vi "P4CMD Dialog - File History.vi"(6 "files":string[](array[string]), 7 "fstat info":string, 8 "error in (no error)":errorcluster, 10 "revision string":string, 11 "source control reference in":T1) -> (0 "error out":errorcluster, 5 "file changed?":bool)   [LabVIEW 2017, in "NI_SCC_P4CMD.lvlib"]
uses:
  <vilib>/SourceControl/Providers/P4CMD/NI_SCC_P4CMD.lvlib
  <vilib>/SourceControl/sccapi/SCCAPI Refnum.ctl
  <vilib>/event_ctls.llb/sizeaction.ctl
  <vilib>/event_ctls.llb/panelstate.ctl
  <vilib>/SourceControl/Providers/P4CMD/P4CMD Operations.ctl
  <vilib>/SourceControl/support/SCCSup Message Strings GLBL.vi
  <vilib>/SourceControl/sccapi/NI_SCC.lvlib
  <vilib>/Utility/lvfile.llb/NI_FileType.lvlib
panel:
  in  "History":i32[](listbox)
  in  "Depot file":i32(ring)
  out "File type:":string
  out "Actions in changelist":string
  out "Description of changelist":string
  in  "OK":bool
  in  "Help":bool
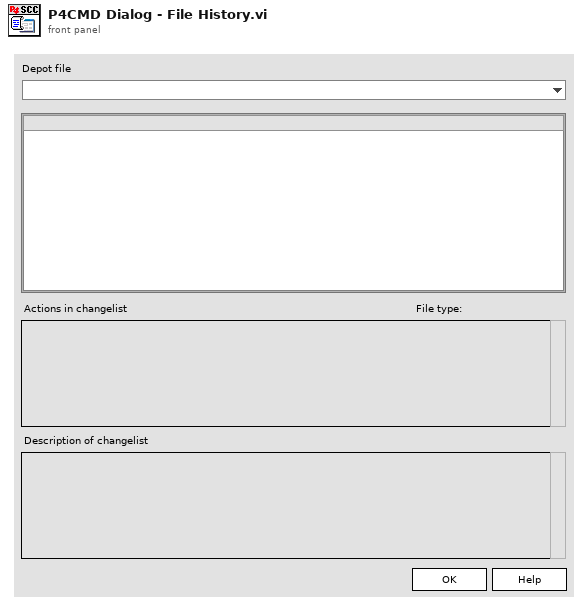
[diagram p1: front panel]
types:
  T1 = typedef "NI_SCC.lvlib/SCCAPI Refnum.ctl" = refnum<k1>
  T2 = enum32{"invalid OS target", "Mac OS", "Windows 3.1", "Windows 95/NT", "Solaris 1", "Solaris 2", "HP-UX", "PowerMAX", "Linux", "Irix", "Rhapsody", "BeOS", "AIX", "OSF1", "VxWorks", "PharLap", "Carbon", "RTX", "Windows x64", "Linux x64"}
  T3 = typedef "sizeaction.ctl" = enum32{"Minimized", "Maximized", "Resized"}
  T4 = typedef "panelstate.ctl" = enum32{"Standard", "Minimized", "Maximized"}
  T5 = typedef "NI_SCC_P4CMD.lvlib/P4CMD Operations.ctl" = enum16{"get all clients", "get all users", "describe changelist", "sync from depot", "open for edit", "submit to depot", "revert", "add to depot", "remove from depot", "print files revisions", "compare client file", "print depot file contents", "list opened files", "get file info", "lock files", "edit changelist spec", "info", "set variables"}
  T6 = enum32{"Invalid", "Standard", "Closed", "Hidden", "Minimized", "Maximized"}
  T7 = typedef "imagedata.ctl" = cluster{"image type":i32, "image depth":i32, "image":u8[], "mask":u8[], "colors":u32[], "Rectangle":cluster{"left":i16, "top":i16, "right":i16, "bottom":i16}}
  T8 = typedef "LVRectTypeDef.ctl" = cluster{"Left":i16, "Top":i16, "Right":i16, "Bottom":i16}
  T9 = enum32{"invalid OS target", "Mac OS", "Windows 3.1", "Windows 95/NT", "Solaris 1", "Solaris 2", "HP-UX", "PowerMAX", "Linux", "Irix", "Rhapsody", "BeOS", "AIX", "OSF1", "VxWorks", "PharLap", "Carbon", "RTX", "Windows x64", "Linux x64", "Mac OS X x64"}
  T10 = typedef "eventvkey.ctl" = enum16{"ASCII", "Enter", "Return", "Shift", "Ctrl", "Alt", "Cmd", "Opt", "Caps", "NumLock", "Clear", "Break", "Up", "Down", "Left", "Right", "Insert", "Delete", "Home", "End", "PageUp", "PageDown", "Escape", "Help", "Pause", "ScrollLock", "F1", "F2", "F3", "F4", "F5", "F6", "F7", "F8", "F9", "F10", "F11", "F12", "F13", "F14", "F15", "F16", "F17", "F18", "F19", "F20", "F21", "F22", "F23", "F24", "Play", "VolumeUp", "VolumeDown", "Mute", "Two Byte Char"}
  T11 = typedef "LVPoint32TypeDef.ctl" = cluster{"Horizontal":i32, "Vertical":i32}
  T12 = typedef "LVRowAndColumnTypeDef.ctl" = cluster{"Row":i32, "Column":i32}
  T13 = typedef "NI_SCC.lvlib/SCCAPI VI Compare Options.ctl" = cluster{"VI Attributes":bool, "Front Panel":bool, "FP position/size":bool, "Block Diagram":bool, "BD cosmetic":bool, "BD position/size":bool}
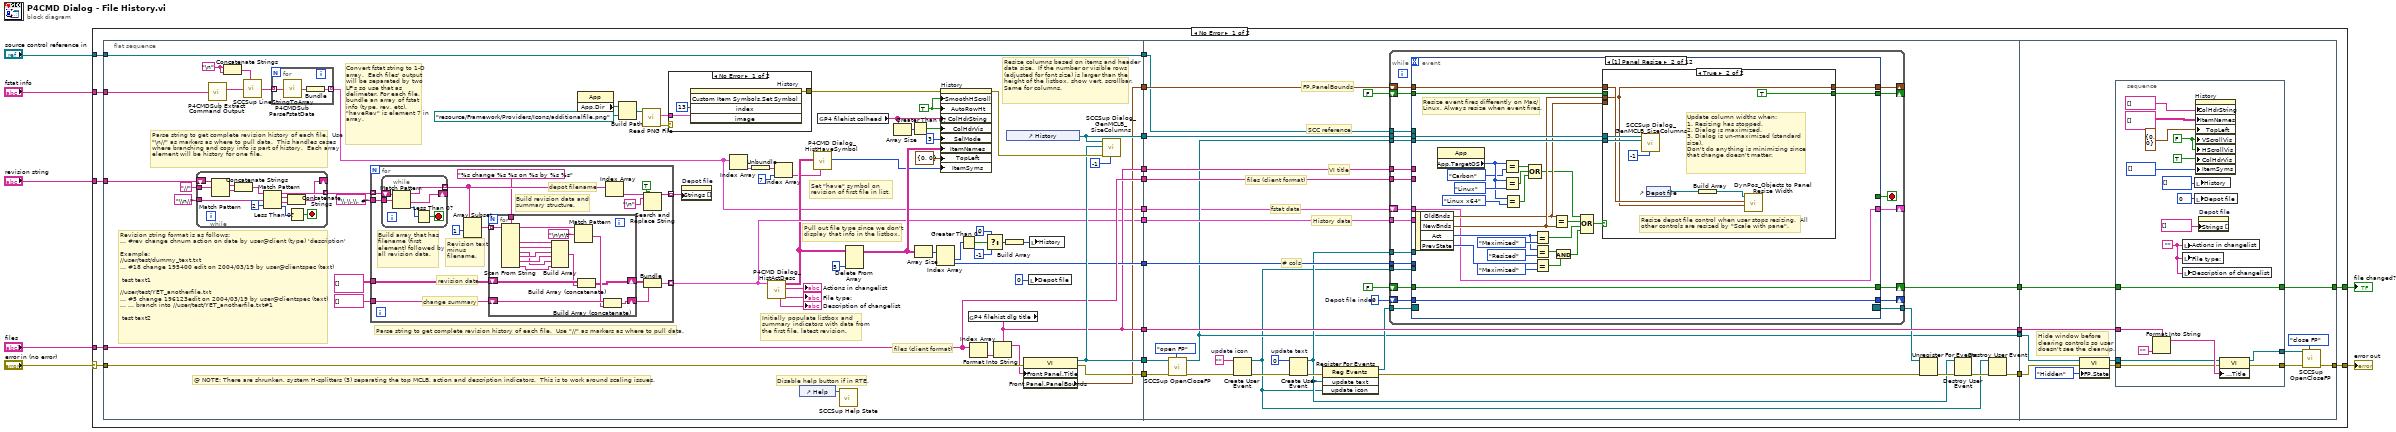
[diagram p0: block diagram]
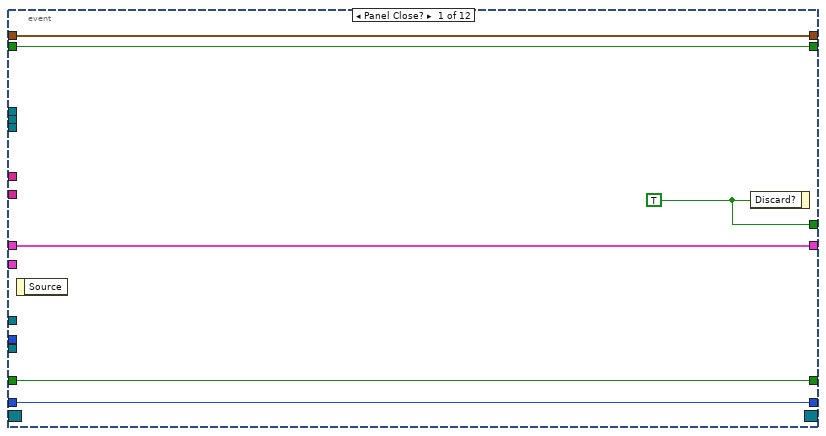
[diagram p3: hidden frame]
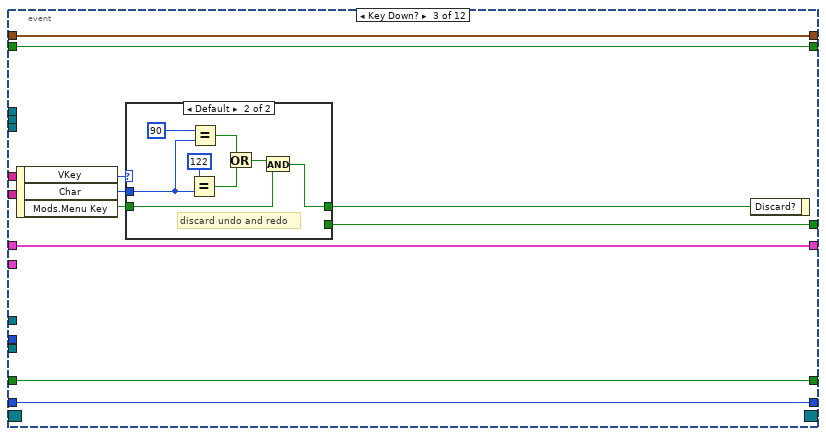
[diagram p6: hidden frame]
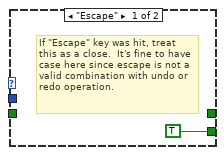
[diagram p7: hidden frame]
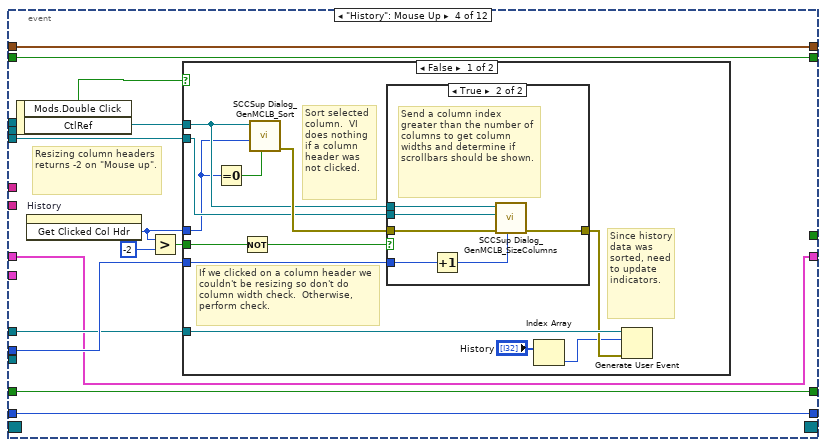
[diagram p8: hidden frame]
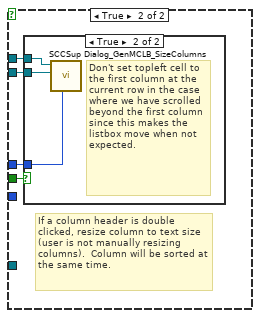
[diagram p10: hidden frame]
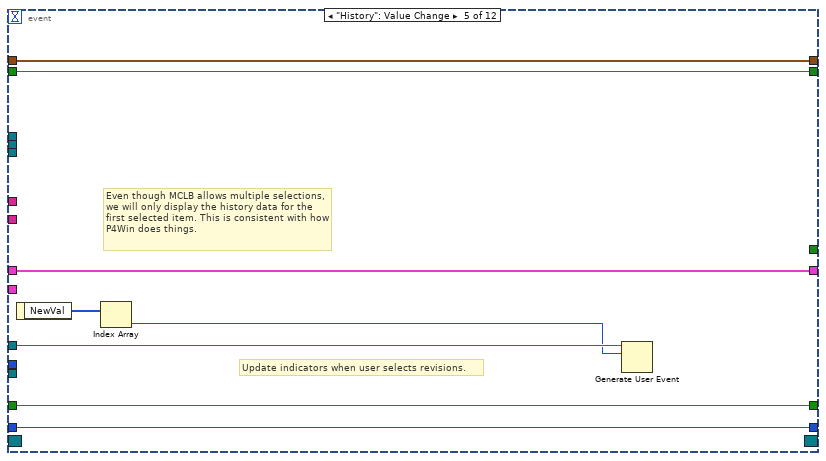
[diagram p12: hidden frame]
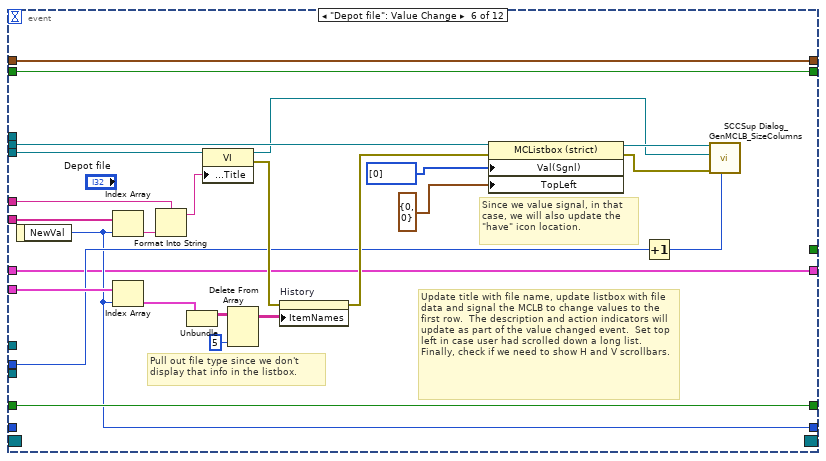
[diagram p13: hidden frame]
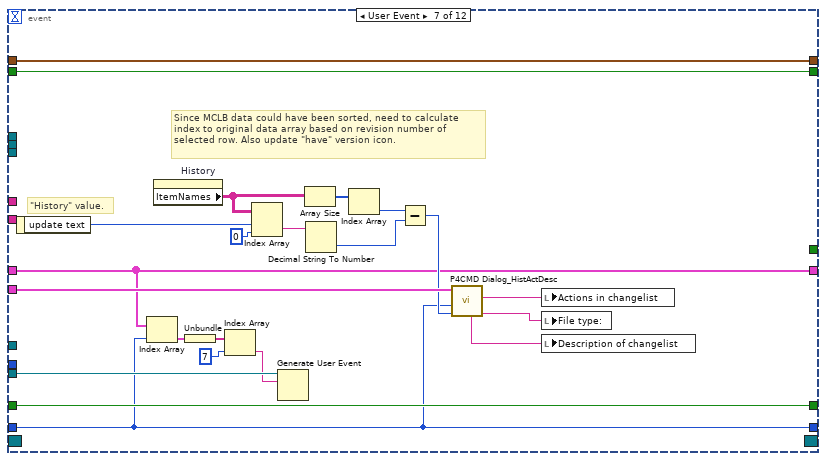
[diagram p14: hidden frame]
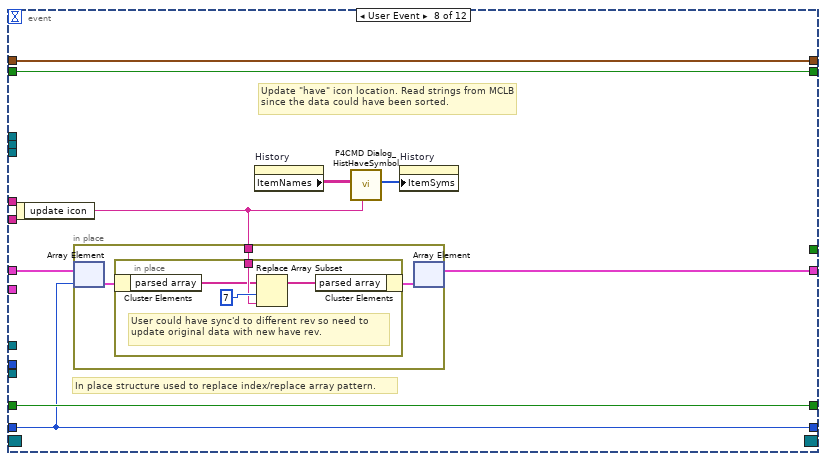
[diagram p15: hidden frame]
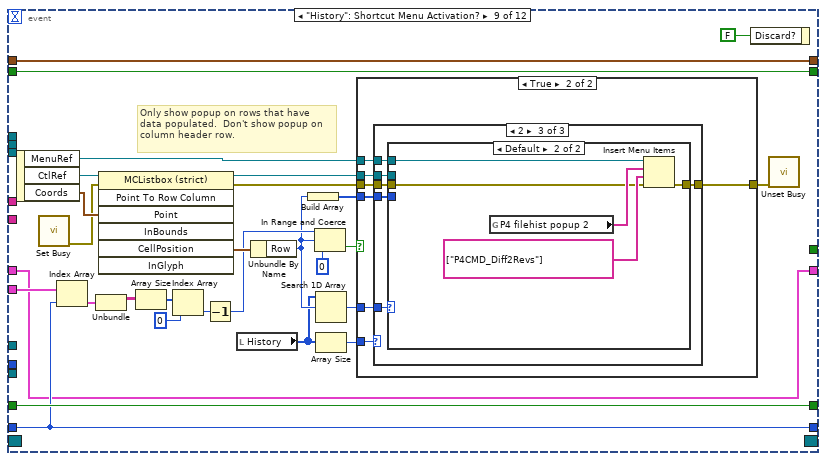
[diagram p16: hidden frame]
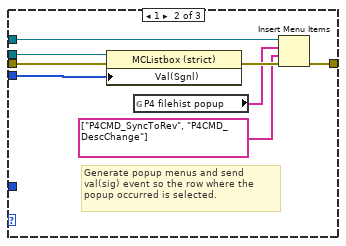
[diagram p19: hidden frame]
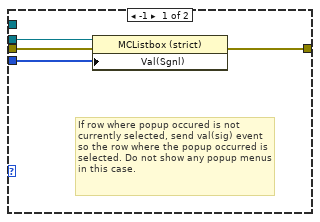
[diagram p20: hidden frame]
diagram:
  n1 = case shown="No Error" "error in (no error)" {
    selector: "error in (no error)" -> [w25 w574]
    tunnel: "revision string" -> [w26 _]
    tunnel: [w22 w574] -> w5
    tunnel: "files" -> [w19 _]
    tunnel: "source control reference in" -> [w13 _]
    tunnel: [w10 _] -> w2
    tunnel: "fstat info" -> [w9 _]
    frame No Error {
      n2 = flat-sequence {
        tunnel: [w82] -> w29
        tunnel: [w83] -> w28
        tunnel: w25 -> [w78]
        tunnel: w26 -> [w60]
        tunnel: [w77] -> w24
        tunnel: [w36] -> w21
        tunnel: [w68] -> w20
        tunnel: w19 -> [w72]
        tunnel: [w72] -> w18
        tunnel: [w64] -> w17
        tunnel: [w64] -> w16
        tunnel: [w56] -> w14
        tunnel: w13 -> [w52]
        tunnel: [w52] -> w12
        tunnel: w9 -> [w39]
        tunnel: [w34] -> w8
        tunnel: [w158] -> w27
        tunnel: w29 -> [w174]
        tunnel: w28 -> [w173]
        tunnel: w24 -> [w172]
        tunnel: [w148] -> w23
        tunnel: w21 -> [w170]
        tunnel: w20 -> [w171]
        tunnel: w18 -> [w169]
        tunnel: w17 -> [w168]
        tunnel: w16 -> [w167]
        tunnel: [w167] -> w15
        tunnel: w14 -> [w166]
        tunnel: w12 -> [w157]
        tunnel: [w155] -> w11
        tunnel: w8 -> [w146]
        tunnel: w27 -> [w549]
        tunnel: w23 -> [w546]
        tunnel: [w551] -> w22
        tunnel: w15 -> [w554]
        tunnel: w11 -> [w545]
        tunnel: [w544] -> w10
        frame #0 {
          w42 = "\n"
          w63 = TRUE ("Smooth Horizontal Scrolling")
          # "Set \"have\" symbol on revision of first file in list."
          # "Revision string format is as follows:\n... #rev change chnum action on date by user@client (type) 'description'\n\nExample:\n//user/test/dummy_text.txt\n... #18 change 195400 edit on 2004/03/19 by user@clientspec (text)\n\n\ttest text1\n\n//user/test/YET_anotherfile.txt\n... #5 change 196123edit on 2004/03/19 by user@clientspec (text)\n... ... branch into //user/test/YET_anotherfile.txt#1\n\n\ttest text2"
          # "Convert fstat string to 1-D array.  Each files' output will be separated by two LF's so use that as delimeter. For each file, bundle an array of fstat info (type, rev, etc). \"haveRev\" is element 7 in array."
          # "@ NOTE: There are shrunken, system H-splitters (3) separating the top MCLB, action and description indicators.  This is to work around scaling issues."
          # "Pull out file type since we don't display that info in the listbox."
          # "Disable help button if in RTE."
          # "files (client format)"
          # "Parse string to get complete revision history of each file.  Use \"//\" as markers as where to pull data."
          # "Parse string to get complete revision history of each file.  Use \"\\n//\" as markers as where to pull data.  This handles cases where branching and copy info is part of history.  Each array element will be history for one file."
          # "Initially populate listbox and summary indicators with data from the first file, latest revision."
          # "Resize columns based on items and header data size.  If the number or visible rows (adjusted for font size) is larger than the height of the listbox, show vert. scrollbar.  Same for columns."
          n3 = while {
            shift-right: [w101] -> _
            shift-left: w60 -> [w107]
            tunnel: "//" ("format string") -> [w105]
            tunnel: [w104] -> w59 mode=indexing
            tunnel: "\\n//" ("format string") -> [w102]
            stop <- w108 stop-if-true
            n4 = Match Pattern(string=w107, regular expression=w105) -> (match substring=w98:string, after substring=w97:string)  [unwired: 1 in, 2 out]
            n5 = Concatenate Strings(w98, w97) -> (w96:string)
            n6 = Match Pattern(string=w96, regular expression=w102, offset (0)=2) -> (before substring=w104:string, match substring=w99:string, after substring=w106:string, offset past match=w100:i32)
            n7 = Concatenate Strings(w99, w106) -> (w101:string)
            n8 = Less Than 0?(x=w100) -> (x < 0?=w108:bool)
          }
          n9 = call <vilib>:"P4CMDSub Extract Command Output.vi"("bundled message"=w39) -> ("command output"=w40:string)  [unwired: 13 in, 1 out]
          n10 = Concatenate Strings(w42, w42) -> (w41:string)
          n11 = call <vilib>:"SCCSup LineStringToArray.vi"("delimiter (Tab)"=w41, "line string"=w40) -> ("line array"=w38:string[])  [unwired: 7 in]
          n12 = for {
            tunnel: w38 -> [w92] mode=indexing
            tunnel: [w90] -> w34 mode=indexing
            n13 = call <vilib>:"P4CMDSub ParseFstatData.vi"("fstat data"=w92) -> ("parsed array"=w91:string[])  [unwired: 4 in]
            n14 = Bundle("parsed array"=w91) -> (w90:cluster{"parsed array":string[]})  [unwired: 1 in]
          }
          n15 = for {
            tunnel: w59 -> [w119] mode=indexing
            tunnel: [w115] -> w75 mode=indexing
            tunnel: "\\.\\.\\. #" ("regular expression") -> [w118]
            tunnel: string[][] [] -> [w114]
            tunnel: string[] [] -> [w113]
            tunnel: [w110] -> w36 mode=indexing
            # "Build revision data and summary structure."
            # "Build array that has filename (first element) followed by all revision data."
            # "Revision text minus filename."
            # "depot filename"
            # "revision data"
            # "change summary"
            n16 = while {
              shift-right: [w125] -> _
              shift-left: w119 -> [w129]
              tunnel: [w128] -> w116 mode=indexing
              tunnel: w118 -> [w124]
              stop <- w127 stop-if-true
              n17 = Match Pattern(string=w129, regular expression=w124) -> (before substring=w128:string, after substring=w125:string, offset past match=w126:i32)  [unwired: 1 in, 1 out]
              n18 = Less Than 0?(x=w126) -> (x < 0?=w127:bool)
            }
            n19 = Array Subset(array=w116, index=1) -> (w122:string[])  [unwired: 1 in]
            n20 = for {
              tunnel: w122 -> [w136] mode=indexing
              shift-right: [w133] -> w112
              shift-left: w114 -> [w145]
              shift-right: [w137] -> w111
              shift-left: w113 -> [w144]
              tunnel: "%s change %s %s on %s by %s %s" ("Format String") -> [w132]
              n21 = Scan From String(format string=w132, input string=w136) -> (remaining string=w131:string, output 1=w143:string, output 2=w142:string, output 3=w138:string, output 4=w140:string, output 5=w139:string, output 6=w130:string)  [unwired: 8 in, 2 out]
              n22 = Build Array(w143, w142, w140, w139, w138, w130) -> (w141:string[])
              n23 = Match Pattern(string=w131, regular expression="\n\n\t") -> (after substring=w134:string)  [unwired: 1 in, 3 out]
              n24 = Build Array (concatenate)(w145, w141) -> (w133:string[][])
              n25 = Build Array (concatenate)(w144, w134) -> (w137:string[])
            }
            n26 = Index Array(array=w116) -> (element=w121:string)  [unwired: 1 in]
            n27 = Search and Replace String(replace all?=TRUE ("replace all? (F)"), input string=w121, search string="\n" ("Line Feed Constant")) -> (result string=w115:string)  [unwired: 5 in, 3 out]
            n28 = Bundle(w112, w111) -> (w110:cluster{string[][], string[]})  [unwired: 1 in]
          }
          n29 = property class="App"() -> ("App.Dir"=w46:path)  [unwired: 2 in, 2 out]
          n30 = Build Path(base path=w46, name or relative path=path "resource/Framework/Providers/Icons/additionalfile.png" ("base path")) -> (appended path=w44:path)
          n31 = call <vilib>:"Read PNG File.vi"("path to PNG file"=w44) -> ("error out"=w43:errorcluster, "image data"=w48:T7)  [unwired: 8 in, 1 out]
          n32 = case shown="No Error" w43 {
            tunnel: [w95 _] -> w49
            tunnel: w48 -> [w94 _]
            frame No Error {
              n33 = invoke on="History" class="MCListbox (strict)" method="Custom Item Symbols.Set Symbol"("index"=13 ("Index"), "image"=w94) -> (error out=w95:errorcluster)  [unwired: 3 in, 4 out]
            }
            frame Error {
              # "If there was a problem reading the custom icon, use default image."
            }
          }
          n34 = property on="Depot file" class="Ring (strict)"("Strings []"=w75) -> ()  [unwired: 2 in, 2 out]
          n35 = Index Array(array=w34) -> (element=w33:cluster{"parsed array":string[]})  [unwired: 1 in]
          n36 = Unbundle(w33) -> ("parsed array"=w32:string[])
          n37 = call <vilib>:"P4CMD Dialog_HistActDesc.vi"("history array"=w36) -> ("file type"=→"File type:":string, "action"=→"Actions in changelist":string, "revision data"=w35:string[][], "description"=→"Description of changelist":string)  [unwired: 7 in]
          n38 = Index Array(array=w32, index=7) -> (element=w30:string)
          n39 = control-ref of="Help"() -> (w58:refnum<vi>)
          n40 = call <vilib>:"P4CMD Dialog_HistHaveSymbol.vi"("have revision"=w30, "history info"=w35) -> ("symbols"=w47:i32[])  [unwired: 9 in]
          n41 = global read "SCCSup Message Strings GLBL.vi" "P4 filehist colhead"() -> (w65:string[])
          n42 = call <vilib>:"SCCSup Help State.vi"("help ref"=w58) -> ()  [unwired: 10 in, 1 out]
          n43 = Delete From Array(array=w35, index (col)=5 ("disabled index (col)")) -> (array with subset deleted=w50:string[][])  [unwired: 2 in, 1 out]
          n44 = Array Size(array=w65) -> (size(s)=w88:i32)
          n45 = Greater Than 0?(x=w88) -> (x > 0?=w66:bool)
          n46 = Array Size(array=w50) -> (size(s)=w69:i32[])
          n47 = Index Array(array=w69) -> (element #1=w51:i32, element #2=w68:i32)  [unwired: 2 in]
          n48 = property on="History" class="MCListbox (strict)"(error in=w49, "SmoothHScroll"=w63, "AutoRowHt"=w63, "ColHdrString"=w65, "ColHdrVis"=w66, "SelMode"=3 ("Selection Mode"), "ItemNames"=w50, "TopLeft"=cluster{"Row":u32, "Column":u32} {"Row"=0, "Column"=0} ("Top Left Visible Cell"), "ItemSyms"=w47) -> (error out=w85:errorcluster)  [unwired: 1 in, 1 out]
          n49 = Greater Than 0?(x=w51) -> (x > 0?=w81:bool)
          n50 = global read "SCCSup Message Strings GLBL.vi" "P4 filehist dlg title"() -> (w64:string)
          n51 = Index Array(array=w72) -> (element=w74:string)  [unwired: 1 in]
          n52 = Select(t=0, s=w81, f=-1 ("index of element")) -> (s? t:f=w89:i32)
          n53 = Format Into String(format string=w64, w74) -> (resulting string=w73:string)  [unwired: 2 in, 1 out]
          n54 = Build Array(w89) -> (w84:i32[])
          n55 = control-ref of="History"() -> (w83:refnum<vi>)
          n56 = property on="Property Node" class="VI"(error in=w78, "Front Panel.Title"=w73) -> (reference out=w82:refnum<vi>, error out=w77:errorcluster, "Front Panel.PanelBounds"=w56:T8)  [unwired: 1 in]
          n57 = local write "Depot file"(0 ("Depot file")) -> ()
          n58 = local write "History"(w84) -> ()
          n59 = call <vilib>:"SCCSup Dialog_GenMCLB_SizeColumns.vi"("column index"=-1, "error in (no error)"=w85, "VI Refnum"=w82, "Multicolumn Listbox"=w83) -> ()  [unwired: 6 in, 2 out]
        }
        frame #1 {
          w152 = ""  # update icon
          w153 = 0  # update text
          w154 = 0  # Depot file index
          # "SCC reference"
          # "# cols"
          # "fstat data"
          # "History data"
          # "VI title"
          # "FP.PanelBounds"
          # "files (client format)"
          n60 = call <vilib>:"SCCSup OpenCloseFP.vi"("function"=enum16{"open FP", "close FP"}."open FP", "error in (no error)"=w172, "VI Refnum in"=w174) -> ("error out"=w150:errorcluster, "VI Refnum out"=w158:refnum<vi>)  [unwired: 7 in]
          n61 = Create User Event(user event datatype=w152, error in=w150) -> (user event=w147:refnum<user-event>, error out=w151:errorcluster)
          n62 = Create User Event(user event datatype=w153, error in=w151) -> (user event=w159:refnum<user-event>, error out=w164:errorcluster)
          n63 = register-events(error in=w164, w159, w147) -> (reference out=w163:refnum<event-registration>, error out=w161:errorcluster)  [unwired: 1 in]
          n64 = while {
            tunnel: w158 -> [w195]
            tunnel: w173 -> [w196]
            tunnel: w171 -> [w194]
            tunnel: w170 -> [w193]
            tunnel: w169 -> [w192]
            tunnel: w168 -> [w191]
            shift-right: [w187] -> _
            shift-left: w166 -> [w190]
            shift-right: [w189] -> _
            shift-left: FALSE -> [w188]
            tunnel: w163 -> [w186]
            tunnel: [w185] -> w162
            tunnel: w159 -> [w184]
            tunnel: w157 -> [w183]
            shift-right: [w181] -> w155
            shift-left: FALSE -> [w182]
            shift-right: [w179] -> _
            shift-left: w154 -> [w180]
            tunnel: w147 -> [w178]
            shift-right: [w176] -> _
            shift-left: w146 -> [w177]
            stop <- w197 stop-if-true
            n65 = event shown="[1] Panel Resize" {
              selector: w186 -> [_ _ _ _ _ _ _ _ _ _ _ _]
              dyn-events: [_ _ _ _ _ _ _ _ _ _ _ _] -> w185
              timeout: _ -> [_ _ _ _ _ _ _ _ _ _ _ _]
              tunnel: [w203 _ w255 _ _ _ _ _ _ w439 "OK" _] -> w197
              tunnel: w196 -> [_ w233 _ _ _ w328 _ _ _ _ _ _]
              tunnel: w195 -> [_ w232 _ w277 _ w338 _ _ _ _ _ _]
              tunnel: w194 -> [_ _ _ w276 _ w319 _ _ _ _ _ _]
              tunnel: w193 -> [_ _ _ _ _ w331 w359 _ w396 _ _ _]
              tunnel: w192 -> [_ _ _ _ _ w339 _ _ _ w453 _ _]
              tunnel: w191 -> [_ _ _ _ _ w336 _ _ _ _ _ _]
              tunnel: w190 -> [w202 w221 w254 w273 w315 w334 w353 w370 w406 w460 w534 w540]
              tunnel: [w201 w218 w253 w274 w314 w333 w352 w369 w405 w459 w533 w539] -> w189
              tunnel: w188 -> [w201 w217 w253 w274 w314 w333 w352 w369 w405 w459 w533 w539]
              tunnel: [w202 w216 w254 w273 w315 w334 w353 w370 w406 w460 w534 w540] -> w187
              tunnel: w184 -> [_ _ _ w272 w313 _ _ _ _ _ _ _]
              tunnel: w183 -> [_ _ _ _ _ _ _ _ _ w448 _ _]
              tunnel: w182 -> [w200 w212 w252 w271 w311 w329 w351 w371 w385 w447 w532 w538]
              tunnel: [w200 w212 w252 w271 w311 w329 w351 w371 w385 w446 w532 w538] -> w181
              tunnel: w180 -> [w199 w211 w251 w270 w310 _ w343 w364 w384 w443 w531 w537]
              tunnel: [w199 w211 w251 w270 w310 w317 w343 w364 w384 w443 w531 w537] -> w179
              tunnel: w178 -> [_ _ _ _ _ _ w348 _ _ w442 _ _]
              tunnel: w177 -> [w198 w210 w250 w269 w308 w316 w341 w365 w383 w441 w530 w536]
              tunnel: [w198 w210 w250 w269 w308 w316 w341 w363 w383 w441 w530 w536] -> w176
              event Panel Close? {
                w203 = TRUE
                n66 = event-data() -> ()  [unwired: 1 in, 1 out]
                n67 = event-data ("Event Filter Node")("Discard?"=w203) -> ()  [unwired: 1 in, 1 out]
              }
              event Panel Resize {
                # "Resize event fires differently on Mac/Linux. Always resize when event fires."
                n68 = event-data() -> ("OldBnds"=w219:T8, "NewBnds"=w220:T8, "Act"=w226:T3, "PrevState"=w228:T4)  [unwired: 1 in]
                n69 = property class="App"() -> ("App.TargetOS"=w207:T9)  [unwired: 2 in, 2 out]
                n70 = Equal?(x=w207, y=T2."Carbon" ("Application:Target:Operating System")) -> (x = y?=w214:bool)
                n71 = Equal?(x=w207, y=T2."Linux" ("Application:Target:Operating System")) -> (x = y?=w208:bool)
                n72 = Equal?(x=w207, y=T2."Linux x64" ("Application:Target:Operating System")) -> (x = y?=w205:bool)
                n73 = Compound Arithmetic op=OR(w214, w208, w205) -> (w213:bool)
                n74 = Equal?(x=w226, y=sizeaction."Maximized") -> (x = y?=w229:bool)
                n75 = Equal?(x=w226, y=sizeaction."Resized") -> (x = y?=w224:bool)
                n76 = Equal?(x=w228, y=panelstate."Maximized" ("PrevState")) -> (x = y?=w223:bool)
                n77 = Equal?(x=w219, y=w220) -> (x = y?=w215:bool)
                n78 = And(x=w224, y=w223) -> (x .and. y?=w222:bool)
                n79 = Compound Arithmetic op=OR(w213, w215, w229, w222) -> (w230:bool)
                n80 = case shown="True" w230 {
                  tunnel: w233 -> [_ w249]
                  tunnel: w232 -> [_ w248]
                  tunnel: w221 -> [w238 w244]
                  tunnel: w220 -> [_ w243]
                  tunnel: w219 -> [w237 _]
                  tunnel: [w236 TRUE] -> w218
                  tunnel: w217 -> [w235 _]
                  tunnel: [w234 w243] -> w216
                  frame False {
                    # "Save panel bound after first resize so when resize stops, we can do a correct delta. Once we get the bounds, just pass value through all cases."
                    n81 = case shown="True" w235 {
                      selector: w235 -> [w240 _]
                      tunnel: w238 -> [w239 _]
                      tunnel: w237 -> [_ w241]
                      tunnel: [w240 _] -> w236
                      tunnel: [w239 w241] -> w234
                      frame False {
                      }
                      frame True {
                      }
                    }
                  }
                  frame True {
                    # "Update column widths when:\n1. Resizing has stopped.\n2. Dialog is maximized.\n3. Dialog is un-maximized (standard size).\nDon't do anything is minimizing since that change doesn't matter."
                    # "Resize depot file control when user stops resizing.  All other controls are resized by \"Scale with pane\"."
                    n82 = call <vilib>:"SCCSup Dialog_GenMCLB_SizeColumns.vi"("column index"=-1, "VI Refnum"=w248, "Multicolumn Listbox"=w249) -> ()  [unwired: 7 in, 2 out]
                    n83 = control-ref of="Depot file"() -> (w245:refnum<vi>)
                    n84 = Build Array(w245) -> (w246:refnum<vi>[])
                    n85 = call <vilib>:"DynPos_Objects to Panel Resize Width.vi"("NewBnds"=w243, "OldBnds"=w244, "GObj Refnums"=w246) -> ()  [unwired: 8 in, 1 out]
                  }
                }
              }
              event Key Down? {
                n86 = event-data() -> ("VKey"=w256:T10, "Char"=w259:i16, "Mods.Menu Key"=w258:bool)  [unwired: 1 in]
                n87 = case shown="Default" w256 {
                  tunnel: w259 -> [_ w263]
                  tunnel: w258 -> [_ w262]
                  tunnel: [_ w261] -> w257
                  tunnel: [TRUE _] -> w255
                  frame "Escape" {
                    # "If \"Escape\" key was hit, treat this as a close.  It's fine to have case here since escape is not a valid combination with undo or redo operation."
                  }
                  frame Default {
                    # "discard undo and redo"
                    n88 = Equal?(x=i16 122, y=w263) -> (x = y?=w266:bool)
                    n89 = Equal?(x=i16 90, y=w263) -> (x = y?=w265:bool)
                    n90 = Or(x=w265, y=w266) -> (x .or. y?=w264:bool)
                    n91 = And(x=w264, y=w262) -> (x .and. y?=w261:bool)
                  }
                }
                n92 = event-data ("Event Filter Node")("Discard?"=w257) -> ()  [unwired: 1 in, 1 out]
              }
              event "History": Mouse Up {
                # "Resizing column headers returns -2 on \"Mouse up\"."
                n93 = event-data() -> ("Mods.Double Click"=w275:bool, "CtlRef"=w281:refnum<vi>)  [unwired: 1 in]
                n94 = invoke on="History" class="MCListbox (strict)" method="Get Clicked Col Hdr"() -> ("Get Clicked Column Header"=w279:i32)  [unwired: 3 in, 2 out]
                n95 = Greater?(x=w279, y=-2) -> (0:w278:bool)
                n96 = case shown="False" w275 {
                  tunnel: w281 -> [w288 w304]
                  tunnel: w279 -> [w283 w303]
                  tunnel: w278 -> [w293 w302]
                  tunnel: w277 -> [w289 w301]
                  tunnel: w276 -> [w291 _]
                  tunnel: w272 -> [w287 _]
                  frame False {
                    # "Since history data was sorted, need to update indicators."
                    # "Sort selected column.  VI does nothing if a column header was not clicked."
                    # "If we clicked on a column header we couldn't be resizing so don't do column width check.  Otherwise, perform check."
                    n97 = Equal To 0?(x=w283) -> (x = 0?=w282:bool)
                    n98 = Not(x=w293) -> (.not. x?=w292:bool)
                    n99 = call <vilib>:"SCCSup Dialog_GenMCLB_Sort.vi"("treat as number?"=w282, "Clicked Col Hdr"=w283, "MCListbox Refnum"=w288) -> ("error out"=w290:errorcluster)  [unwired: 8 in]
                    n100 = case shown="True" w292 {
                      tunnel: w288 -> [_ w300]
                      tunnel: w289 -> [_ w299]
                      tunnel: w291 -> [_ w297]
                      tunnel: w290 -> [w294 w296]
                      tunnel: [w294 w295] -> w286
                      frame False {
                      }
                      frame True {
                        # "Send a column index greater than the number of columns to get column widths and determine if scrollbars should be shown."
                        n101 = Increment(x=w297) -> (x+1=w298:i32)
                        n102 = call <vilib>:"SCCSup Dialog_GenMCLB_SizeColumns.vi"("column index"=w298, "error in (no error)"=w296, "VI Refnum"=w299, "Multicolumn Listbox"=w300) -> ("error out"=w295:errorcluster)  [unwired: 6 in, 1 out]
                      }
                    }
                    n103 = Index Array(array="History") -> (element=w284:i32)  [unwired: 1 in]
                    n104 = Generate User Event(user event=w287, event data cluster=w284, error in=w286) -> ()  [unwired: 1 in, 2 out]
                  }
                  frame True {
                    # "If a column header is double clicked, resize column to text size (user is not manually resizing columns).  Column will be sorted at the same time."
                    n105 = case shown="True" w302 {
                      tunnel: w303 -> [_ w307]
                      tunnel: w304 -> [_ w306]
                      tunnel: w301 -> [_ w305]
                      frame False {
                      }
                      frame True {
                        # "Don't set topleft cell to the first column at the current row in the case where we have scrolled beyond the first column since this makes the listbox move when not expected."
                        n106 = call <vilib>:"SCCSup Dialog_GenMCLB_SizeColumns.vi"("column index"=w307, "VI Refnum"=w305, "Multicolumn Listbox"=w306) -> ()  [unwired: 7 in, 2 out]
                      }
                    }
                  }
                }
              }
              event "History": Value Change {
                # "Even though MCLB allows multiple selections, we will only display the history data for the first selected item. This is consistent with how P4Win does things."
                # "Update indicators when user selects revisions."
                n107 = event-data() -> ("NewVal"=w312:i32[])  [unwired: 1 in]
                n108 = Index Array(array=w312) -> (element=w309:i32)  [unwired: 1 in]
                n109 = Generate User Event(user event=w313, event data cluster=w309) -> ()  [unwired: 2 in, 2 out]
              }
              event "Depot file": Value Change {
                # "Since we value signal, in that case, we will also update the \"have\" icon location."
                # "Pull out file type since we don't display that info in the listbox."
                # "Update title with file name, update listbox with file data and signal the MCLB to change values to the first row.  The description and action indicators will update as part of the value changed event.  Set top left in case user had scrolled down a long list. Finally, check if we need to show H and V scrollbars."
                n110 = event-data() -> ("NewVal"=w317:i32)  [unwired: 1 in]
                n111 = Index Array(array=w339, index=w317) -> (element=w340:string)
                n112 = Index Array(array=w331, index=w317) -> (element=w332:cluster{string[][], string[]})
                n113 = Format Into String(format string=w336, w340) -> (resulting string=w337:string)  [unwired: 2 in, 1 out]
                n114 = Unbundle(w332) -> (w330:string[][])  [unwired: 1 out]
                n115 = property on="Property Node" class="VI"(reference=w338, "Front Panel.Title"=w337) -> (reference out=w320:refnum<vi>, error out=w325:errorcluster)  [unwired: 1 in]
                n116 = Delete From Array(array=w330, index (col)=5 ("disabled index (col)")) -> (array with subset deleted=w318:string[][])  [unwired: 2 in, 1 out]
                n117 = property on="History" class="MCListbox (strict)"(error in=w325, "ItemNames"=w318) -> (error out=w326:errorcluster)  [unwired: 1 in, 1 out]
                n118 = property on="Property Node" class="MCListbox (strict)"(reference=w328, error in=w326, "Val(Sgnl)"=i32[] [0] ("History"), "TopLeft"=cluster{"Row":u32, "Column":u32} {"Row"=0, "Column"=0} ("Top Left Visible Cell")) -> (reference out=w322:refnum<vi>, error out=w321:errorcluster)
                n119 = Increment(x=w319) -> (x+1=w323:i32)
                n120 = call <vilib>:"SCCSup Dialog_GenMCLB_SizeColumns.vi"("column index"=w323, "error in (no error)"=w321, "VI Refnum"=w320, "Multicolumn Listbox"=w322) -> ()  [unwired: 6 in, 2 out]
              }
              event User Event {
                # "\"History\" value."
                # "Since MCLB data could have been sorted, need to calculate index to original data array based on revision number of selected row. Also update \"have\" version icon."
                n121 = event-data() -> ("update text"=w354:i32)  [unwired: 1 in]
                n122 = Index Array(array=w341, index=w343) -> (element=w346:cluster{"parsed array":string[]})
                n123 = property on="History" class="MCListbox (strict)"() -> ("ItemNames"=w350:string[][])  [unwired: 2 in, 2 out]
                n124 = Unbundle(w346) -> ("parsed array"=w345:string[])
                n125 = Index Array(array=w345, index=7) -> (element=w342:string)
                n126 = Index Array(array=w350, index (row)=w354, index (col)=0 ("disabled index (col)")) -> (element=w357:string)
                n127 = Generate User Event(user event=w348, event data cluster=w342) -> ()  [unwired: 2 in, 2 out]
                n128 = Array Size(array=w350) -> (size(s)=w356:i32[])
                n129 = Decimal String To Number(string=w357) -> (number=w355:i32)  [unwired: 2 in, 1 out]
                n130 = Index Array(array=w356) -> (element=w349:i32)  [unwired: 1 in]
                n131 = Subtract(x=w349, y=w355) -> (x-y=w347:i32)
                n132 = call <vilib>:"P4CMD Dialog_HistActDesc.vi"("revision index (0)"=w347, "depot file index (0)"=w343, "history array"=w359) -> ("file type"=w361:string, "action"=w362:string, "description"=w360:string)  [unwired: 5 in, 1 out]
                n133 = local write "Actions in changelist"(w362) -> ()
                n134 = local write "File type:"(w361) -> ()
                n135 = local write "Description of changelist"(w360) -> ()
              }
              event User Event {
                # "In place structure used to replace index/replace array pattern."
                # "Update \"have\" icon location. Read strings from MCLB since the data could have been sorted."
                n136 = event-data() -> ("update icon"=w366:string)  [unwired: 1 in]
                n137 = in-place {
                  in-place-border: w366 -> [w374]
                  n138 = in-place-array #1(w365, w364) -> (w373:cluster{"parsed array":string[]})
                  n139 = in-place {
                    in-place-border: w374 -> [w377]
                    # "User could have sync'd to different rev so need to update original data with new have rev."
                    n140 = in-place-cluster #2(w373) -> ("parsed array"=w376:string[])
                    n141 = Replace Array Subset(array=w376, new element=w377, index=7) -> (w375:string[])
                    n142 = in-place-cluster #2("parsed array"=w375) -> (w372:cluster{"parsed array":string[]})
                  }
                  n143 = in-place-array #1(w372) -> (w363:cluster{"parsed array":string[]}[])  [unwired: 1 out]
                }
                n144 = property on="History" class="MCListbox (strict)"() -> ("ItemNames"=w367:string[][])  [unwired: 2 in, 2 out]
                n145 = call <vilib>:"P4CMD Dialog_HistHaveSymbol.vi"("have revision"=w366, "history info"=w367) -> ("symbols"=w368:i32[])  [unwired: 9 in]
                n146 = property on="History" class="MCListbox (strict)"("ItemSyms"=w368) -> ()  [unwired: 2 in, 2 out]
              }
              event "History": Shortcut Menu Activation? {
                # "Only show popup on rows that have data populated.  Don't show popup on column header row."
                n147 = event-data() -> ("MenuRef"=w389:refnum<k9>, "CtlRef"=w404:refnum<vi>, "Coords"=w403:T11)  [unwired: 1 in]
                n148 = call <vilib>:"Set Busy.vi"() -> ("error out"=w402:errorcluster)  [unwired: 10 in, 1 out]
                n149 = Index Array(array=w396, index=w384) -> (element=w401:cluster{string[][], string[]})
                n150 = Unbundle(w401) -> (w400:string[][])  [unwired: 1 out]
                n151 = invoke class="MCListbox (strict)" method="Point To Row Column"(reference=w404, error in=w402, "Point"=w403) -> (reference out=w390:refnum<vi>, error out=w391:errorcluster, "CellPosition"=w395:T12)  [unwired: 4 in, 4 out]
                n152 = Array Size(array=w400) -> (size(s)=w399:i32[])
                n153 = Index Array(array=w399, index=0) -> (element=w398:i32)
                n154 = Decrement(x=w398) -> (x-1=w394:i32)
                n155 = local read "History"() -> (w380:i32[])
                n156 = Unbundle By Name(w395) -> ("Row"=w381:i32)
                n157 = Build Array(w381) -> (w388:i32[])
                n158 = In Range and Coerce(upper limit=w394, x=w381, lower limit=0 ("upper limit")) -> (In Range?=w392:bool)  [unwired: 1 out]
                n159 = Search 1D Array(1D array=w380, element=w381) -> (index of element=w379:i32)  [unwired: 1 in]
                n160 = Array Size(array=w380) -> (size(s)=w382:i32)
                n161 = case shown="True" w392 {
                  tunnel: w391 -> [w407 w414]
                  tunnel: w390 -> [_ w413]
                  tunnel: w389 -> [_ w411]
                  tunnel: w388 -> [_ w412]
                  tunnel: [w407 w410] -> w387
                  tunnel: w382 -> [_ w409]
                  tunnel: w379 -> [_ w408]
                  frame False {
                  }
                  frame True {
                    n162 = case shown="2" w409 {
                      tunnel: w414 -> [w415 w423 w427]
                      tunnel: w413 -> [_ w422 w425]
                      tunnel: w412 -> [_ w421 w424]
                      tunnel: w411 -> [_ w420 w429]
                      tunnel: [w415 w418 w428] -> w410
                      tunnel: w408 -> [_ _ w426]
                      frame 0, Default {
                      }
                      frame 1 {
                        # "Generate popup menus and send val(sig) event so the row where the popup occurred is selected."
                        n163 = property class="MCListbox (strict)"(reference=w422, error in=w423, "Val(Sgnl)"=w421) -> (error out=w419:errorcluster)  [unwired: 1 out]
                        n164 = global read "SCCSup Message Strings GLBL.vi" "P4 filehist popup"() -> (w416:string[])
                        n165 = Insert Menu Items(6:w419, 7:string[] ["P4CMD_SyncToRev", "P4CMD_DescChange"] ("item names"), 8:w416, 9:w420) -> (0:w418:errorcluster)  [unwired: 2 in, 2 out]
                      }
                      frame 2 {
                        n166 = case shown="Default" w426 {
                          tunnel: w429 -> [_ w438]
                          tunnel: [w430 w437] -> w428
                          tunnel: w427 -> [w432 w434]
                          tunnel: w425 -> [w433 _]
                          tunnel: w424 -> [w431 _]
                          frame -1 {
                            # "If row where popup occured is not currently selected, send val(sig) event so the row where the popup occurred is selected. Do not show any popup menus in this case."
                            n167 = property class="MCListbox (strict)"(reference=w433, error in=w432, "Val(Sgnl)"=w431) -> (error out=w430:errorcluster)  [unwired: 1 out]
                          }
                          frame Default {
                            n168 = global read "SCCSup Message Strings GLBL.vi" "P4 filehist popup 2"() -> (w435:string[])
                            n169 = Insert Menu Items(6:w434, 7:string[] ["P4CMD_Diff2Revs"] ("item names"), 8:w435, 9:w438) -> (0:w437:errorcluster)  [unwired: 2 in, 2 out]
                          }
                        }
                      }
                    }
                  }
                }
                n170 = event-data("Discard?"=FALSE) -> ()  [unwired: 1 in, 1 out]
                n171 = call <vilib>:"Unset Busy.vi"("error in (no error)"=w387) -> ()  [unwired: 10 in, 1 out]
              }
              event "History": Shortcut Menu Selection (User) {
                # "Display any errors.  Error is not fatal to this dialog, so we continue."
                n172 = event-data() -> ("ItemTag"=w454:string, "CtlRef"=w458:refnum<vi>, "Coords"=w457:T11)  [unwired: 1 in]
                n173 = call <vilib>:"Set Busy.vi"() -> ("error out"=w456:errorcluster)  [unwired: 10 in, 1 out]
                n174 = invoke class="MCListbox (strict)" method="Point To Row Column"(reference=w458, error in=w456, "Point"=w457) -> (error out=w450:errorcluster, "CellPosition"=w455:T12)  [unwired: 4 in, 5 out]
                n175 = for {
                  tunnel: w453 -> [w462] mode=indexing
                  tunnel: [w461] -> w449 mode=indexing
                  n176 = call <vilib>:"Command Line String To Path.vi"("string"=w462) -> ("path"=w461:path)
                }
                n177 = property on="History" class="MCListbox (strict)"(error in=w450) -> ("ItemNames"=w452:string[][])  [unwired: 1 in, 2 out]
                n178 = Unbundle By Name(w455) -> ("Row"=w451:i32)
                n179 = local read "History"() -> (w440:i32[])
                n180 = case shown="\"P4CMD_Diff2Revs\"" w454 {
                  tunnel: w452 -> [w472 w479 w497]
                  tunnel: w451 -> [w471 w475 _]
                  tunnel: w449 -> [w468 w484 w499]
                  tunnel: [w463 w478 w498] -> w445
                  tunnel: w448 -> [w467 w481 w501]
                  tunnel: w447 -> [w466 _ w502]
                  tunnel: [w466 TRUE w502] -> w446
                  tunnel: w443 -> [_ w477 w500]
                  tunnel: w442 -> [_ w476 _]
                  tunnel: w440 -> [_ _ w496]
                  tunnel: [_ _ w491] -> w439
                  frame "P4CMD_DescChange", Default {
                    # "Files input (and even SCC ref) is not needed, but wire anyway."
                    n181 = Index Array(array=w472, index (row)=w471, index (col)=1 ("disabled index (col)")) -> (element=w469:string)
                    n182 = call <vilib>:"P4CMD Execute Command.vi"("optional operation parameters"=w469, "p4 operation"=P4CMD_Operations."describe changelist", "files"=w468, "source control reference in"=w467) -> ("error out"=w464:errorcluster, "command information"=w465:string)  [unwired: 5 in, 1 out]
                    n183 = call <vilib>:"P4CMD Dialog_HistDispChangelist.vi"("error in (no error)"=w464, "changelist description"=w465) -> ("error out"=w463:errorcluster)  [unwired: 9 in]
                  }
                  frame "P4CMD_SyncToRev" {
                    # "Since we force a sync during a get, notify user that file may have changed."
                    # "Get currently active depot file's client representation at selected revision."
                    n184 = Index Array(array=w479, index (row)=w475, index (col)=0 ("disabled index (col)")) -> (element=w474:string)
                    n185 = Concatenate Strings("#" ("string"), w474) -> (w486:string)
                    n186 = Array Subset(array=w484, index=w477, length=1) -> (w483:path[])
                    n187 = Build Array(w486) -> (w482:string[])
                    n188 = call <vilib>:"P4CMD Get Latest Version.vi"("versions"=w482, "files"=w483, "source control reference in"=w481) -> ("error out"=w478:errorcluster)  [unwired: 5 in, 3 out]
                    n189 = case shown="No Error" w478 {
                      tunnel: w476 -> [w490 _]
                      tunnel: w474 -> [w489 _]
                      frame No Error {
                        # "Since we successfully sync'd to a version, update \"have\" icon location."
                        n190 = Generate User Event(user event=w490, event data cluster=w489) -> ()  [unwired: 2 in, 2 out]
                      }
                      frame Error {
                      }
                    }
                  }
                  frame "P4CMD_Diff2Revs" {
                    n191 = Index Array(array=w499, index=w500) -> (element=w493:path)
                    n192 = Index Array(array=w496) -> (element #1=w495:i32, element #2=w494:i32)  [unwired: 2 in]
                    n193 = call <vilib>:"Is File VI.vi"("path"=w493) -> ("Is VI?"=w492:bool)  [unwired: 8 in, 2 out]
                    n194 = case shown="True" w492 {
                      tunnel: w501 -> [_ w519]
                      tunnel: [_ w514] -> w498
                      tunnel: w497 -> [_ w513]
                      tunnel: w495 -> [_ w512]
                      tunnel: w494 -> [_ w511]
                      tunnel: w493 -> [_ w505]
                      tunnel: [_ w504] -> w491
                      frame False {
                        # "If file is an LLB, we can't compare since SCC API call expects a path to a VI.\nAlso, can't compare non-VIs because Perforce's command line calls are limited when trying to diff text files."
                        n195 = global read "SCCSup Message Strings GLBL.vi" "P4 filehist diff err"() -> (w503:string)
                        n196 = One Button Dialog(message=w503) -> ()  [unwired: 1 in, 1 out]
                      }
                      frame True {
                        w510 = 0 ("disabled index (col)")
                        # "Use MAI to compare since we don't pass a context in. Because this dialog is modal but the compared VIs may not be, we need to close this dialog when comparing."
                        n197 = Index Array(array=w513, index (row) #1=w512, index (col) #1=w510, index (row) #2=w511, index (col) #2=w510) -> (element #1=w507:string, element #2=w506:string)
                        n198 = property class="App"() -> ("App.DefaultApplication"=w515:refnum<vi>)  [unwired: 2 in, 2 out]
                        n199 = Format Into String(format string="#%s,#%s", w507, w506) -> (resulting string=w508:string)  [unwired: 2 in, 1 out]
                        n200 = call <vilib>:"SCCSup Dialog - Compare VIs.vi"() -> ("error out"=w518:errorcluster, "cancelled?"=w516:bool, "compare options out"=w517:T13)  [unwired: 9 in]
                        n201 = case shown="False" w516 {
                          tunnel: w519 -> [w528 _]
                          tunnel: w518 -> [w526 w529]
                          tunnel: w517 -> [w525 _]
                          tunnel: w515 -> [w524 _]
                          tunnel: w505 -> [w523 _]
                          tunnel: [w522 w529] -> w514
                          tunnel: w508 -> [w521 _]
                          tunnel: [TRUE ("interactive? (F)") _] -> w504
                          frame False {
                            n202 = call <vilib>:"SCC Compare VIs.vi"("version"=w521, "interactive? (F)"=TRUE, "application reference"=w524, "error in (no error)"=w526, "compare options"=w525, "VI path"=w523, "source control reference in"=w528) -> ("error out"=w522:errorcluster)  [unwired: 1 in, 3 out]
                          }
                          frame True {
                          }
                        }
                        n203 = Close Reference(reference=w515, error in (no error)=w514) -> ()  [unwired: 1 out]
                      }
                    }
                  }
                }
                n204 = call <vilib>:"SCCSup_Dynam GenErrorHandler.vi"("error in (no error)"=w445) -> ("error out"=w444:errorcluster)  [unwired: 9 in, 1 out]
                n205 = call <vilib>:"Unset Busy.vi"("error in (no error)"=w444) -> ()  [unwired: 10 in, 1 out]
              }
              event "OK": Value Change {
                n206 = event-data() -> ()  [unwired: 1 in, 1 out]
              }
              event "Help": Value Change {
                n207 = event-data() -> ()  [unwired: 1 in, 1 out]
                n208 = call <helpdir>:"_LaunchHelp.vi"("HTML filename"="Perforce_File_History_DB.html" ("Help topic")) -> ("error out"=w542:errorcluster)  [unwired: 6 in]
                n209 = case shown="Error" w542 {
                  selector: w542 -> [_ w543]
                  frame No Error {
                  }
                  frame Error {
                    n210 = call <vilib>:"General Error Handler.vi"("error in (no error)"=w543) -> ()  [unwired: 10 in, 5 out]
                  }
                }
              }
            }
          }
          n211 = Unregister For Events(event registration refnum=w162, error in=w161) -> (error out=w160:errorcluster)
          n212 = Destroy User Event(user event=w159, error in=w160) -> (error out=w149:errorcluster)
          n213 = Destroy User Event(user event=w147, error in=w149) -> (error out=w148:errorcluster)
        }
        frame #2 {
          # "Hide window before clearing controls so user doesn't see the cleanup."
          n214 = property on="Property Node" class="VI"(reference=w549, error in=w546, "FP.State"=T6."Hidden" ("Front Panel Window:State")) -> (reference out=w548:refnum<vi>, error out=w547:errorcluster)
          n215 = stacked-sequence {
            tunnel: w554 -> [w573]
            tunnel: w548 -> [w570]
            tunnel: w547 -> [w569]
            tunnel: [w568] -> w553
            tunnel: [w567] -> w552
            tunnel: w545 -> [w557]
            tunnel: [w557] -> w544
            frame #0 {
              w558 = "" ("Empty String Constant")
              w560 = u16 0 items=[""] ("File")
              w563 = FALSE ("Vertical Scrollbar Visible")
              n216 = Format Into String(format string=w573, "" ("Empty String Constant")) -> (resulting string=w572:string)  [unwired: 2 in, 1 out]
              n217 = local write "Actions in changelist"(w558) -> ()
              n218 = local write "File type:"(w558) -> ()
              n219 = local write "Description of changelist"(w558) -> ()
              n220 = local write "History"(i32[] [] ("MC Listbox")) -> ()
              n221 = local write "Depot file"(w560) -> ()
              n222 = property on="History" class="MCListbox (strict)"("ColHdrString"=string[] [] ("Column Header Strings"), "ItemNames"=string[][] [] ("Item Names"), "TopLeft"=cluster{"Row":u32, "Column":u32} {"Row"=0, "Column"=0} ("Top Left Visible Cell"), "VScrollVis"=w563, "HScrollVis"=w563, "ColHdrVis"=TRUE ("Column Headers Visible"), "ItemSyms"=i32[] [] ("Item Symbols")) -> ()  [unwired: 2 in, 2 out]
              n223 = property on="Depot file" class="Ring (strict)"("Strings []"=string[] []) -> ()  [unwired: 2 in, 2 out]
              n224 = property on="Property Node" class="VI"(reference=w570, error in=w569, "Front Panel.Title"=w572) -> (reference out=w568:refnum<vi>, error out=w567:errorcluster)
            }
          }
          n225 = call <vilib>:"SCCSup OpenCloseFP.vi"("function"=enum16{"open FP", "close FP"}."close FP", "error in (no error)"=w552, "VI Refnum in"=w553) -> ("error out"=w551:errorcluster)  [unwired: 7 in, 1 out]
        }
      }
    }
    frame Error {
    }
  }
  "error out" <- w5
  "file changed?" <- w2
